vi "显示测试结果-取料点相对拍照点移动量.vi"(9 "当前取料点(XY为需要再移动量，ZR为实际值)":T1, 11 "Img输入":T2) -> ()   [LabVIEW 2014]
uses:
  <vilib>/vision/Image Controls.llb/IMAQ Image.ctl
  Controls/XYZRPos.ctl
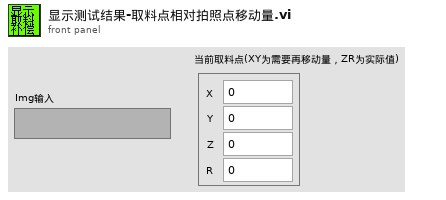
[diagram p1: front panel]
types:
  T1 = typedef "XYZRPos.ctl" = cluster{"X":dbl, "Y":dbl, "Z":dbl, "R":dbl}
  T2 = typedef "IMAQ Image.ctl" = refnum<image>
  T3 = cluster{"Desired Font (Application)":enum16{"User-specified Font", "Application Font", "System Font", "Dialog Font"}, "[User-specified Font]":cluster{"Font Name":string, "Size":i16, "Strikeout?":bool, "Italic?":bool, "Underline?":bool, "Outline?":bool, "Shadow?":bool, "Bold?":bool, "Rotation Angle":dbl}, "Horizontal Alignment":i16, "Vertical Alignment":i16}
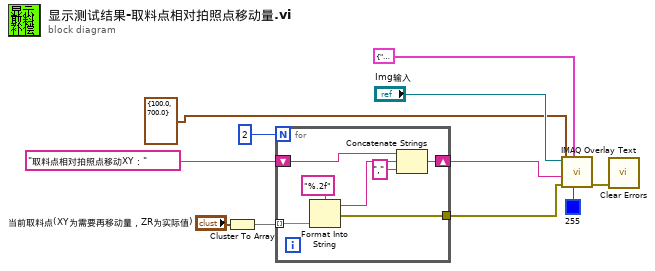
[diagram p0: block diagram]
diagram:
  n1 = Cluster To Array(cluster="当前取料点(XY为需要再移动量，ZR为实际值)") -> (array=w2:dbl[])
  n2 = for {
    N: 2 -> [_]
    tunnel: [w16] -> w7
    shift-right: [w15] -> w5
    shift-left: "取料点相对拍照点移动XY：" -> [w18]
    tunnel: w2 -> [w12] mode=indexing
    n3 = Format Into String(format string="%.2f" ("格式字符串"), w12) -> (resulting string=w14:string, error out=w16:errorcluster)  [unwired: 2 in]
    n4 = Concatenate Strings(w18, w14, "," ("字符串")) -> (w15:string)
  }
  n5 = call "IMAQ Overlay Text"("Text Color (black)"=u32 255, "Font, Size & Style"=T3 {"Desired Font (Application)"=enum."User-specified Font", "[User-specified Font]"={"Font Name"="", "Size"=60, "Strikeout?"=FALSE, "Italic?"=FALSE, "Underline?"=FALSE, "Outline?"=FALSE, "Shadow?"=FALSE, "Bold?"=FALSE, "Rotation Angle"=0.0}, "Horizontal Alignment"=0, "Vertical Alignment"=0}, "error in (no error)"=w7, "String"=w5, "Origin"=cluster{dbl, "Numeric":dbl} {100.0, "Numeric"=700.0}, "Image"="Img输入") -> ("error out"=w6:errorcluster)  [unwired: 4 in, 1 out]
  n6 = call <vilib>:"Clear Errors.vi"("error in (no error)"=w6) -> ()  [unwired: 5 in, 2 out]
